vi "NewPower_Current.vi"(7 "testCurrent":dbl, 8 "error in":errorcluster, 9 "Language":T1, 10 "pwrSwitch":refnum<k21>="Power", 11 "power485":refnum<visa-resource-name>="COM3") -> (0 "error out":errorcluster, 1 "switch":bool[](array[boolean]), 2 "Message":string)   [LabVIEW 2015]
doc: "电源地址\n300A大电源，A002\n5A小电源，A001"
uses:
  CustomControl/Lang_Control.ctl
  <vilib>/DAQmx/write.llb/DAQmx Write (Digital 1D Bool NChan 1Samp 1Line).vi
  <vilib>/Instr/_visa.llb/VISA Configure Serial Port (Instr).vi
  <vilib>/DAQmx/miscellaneous.llb/DAQmx Fill In Error Info.vi
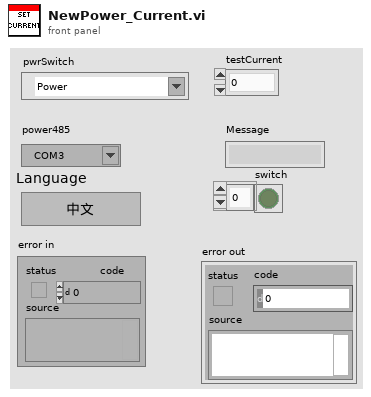
[diagram p1: front panel]
types:
  T1 = typedef "Lang_Control.ctl" = enum16{"中文", "English"}
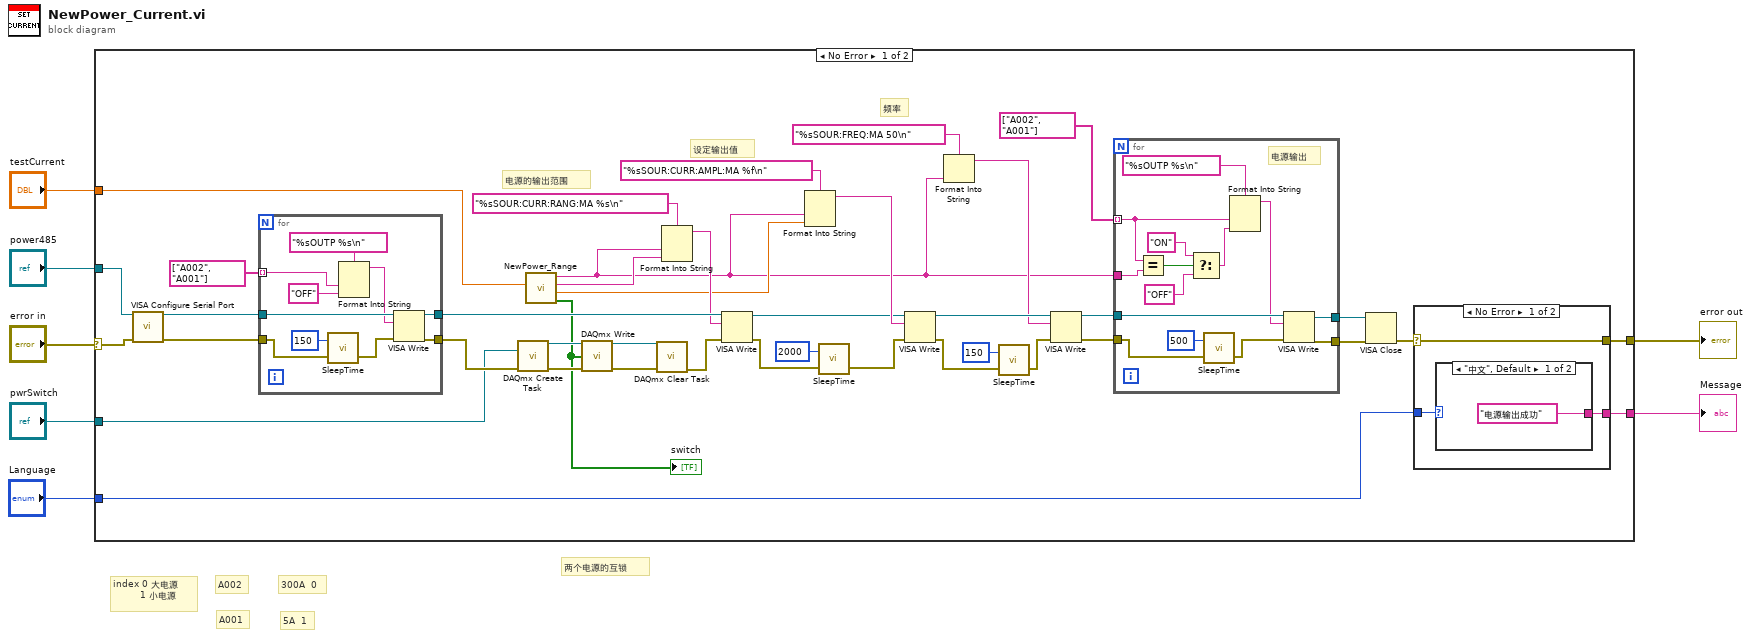
[diagram p0: block diagram]
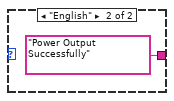
[diagram p2: hidden frame]
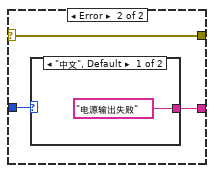
[diagram p3: hidden frame]
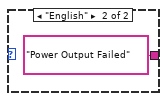
[diagram p4: hidden frame]
diagram:
  # "两个电源的互锁"
  # "index 0 大电源\n         1 小电源"
  # "A001"
  # "A002"
  # "5A  1"
  # "300A  0"
  n1 = case shown="No Error" "error in" {
    selector: "error in" -> [w19 w83]
    tunnel: "power485" -> [w48 _]
    tunnel: "testCurrent" -> [w46 _]
    tunnel: "pwrSwitch" -> [w20 _]
    tunnel: [w17 w83] -> w4
    tunnel: "Language" -> [w16 _]
    tunnel: [w15 _] -> w1
    frame No Error {
      # "频率"
      # "设定输出值"
      # "电源的输出范围"
      n2 = call-poly "VISA Configure Serial Port"("VISA resource name"=w48, "error in (no error)"=w19) -> ("VISA resource name out"=w34:refnum<visa-resource-name>, "error out"=w33:errorcluster)  [unwired: 12 in]
      n3 = for {
        tunnel: w34 -> [w68]
        tunnel: [w67] -> w23
        tunnel: w33 -> [w60]
        tunnel: [w66] -> w32
        tunnel: string[] ["A002", "A001"] -> [w62] mode=indexing
        n4 = call "SleepTime.vi"("error in (no error)"=w60, "Sleep"=u32 150) -> ("error out"=w61:errorcluster)  [unwired: 1 in]
        n5 = Format Into String(format string="%sOUTP %s\n", w62, "OFF" ("format string")) -> (resulting string=w63:string)  [unwired: 2 in, 1 out]
        n6 = VISA Write(VISA resource name=w68, write buffer=w63, error in (no error)=w61) -> (VISA resource name out=w66:refnum<visa-resource-name>, error out=w67:errorcluster)  [unwired: 1 out]
      }
      n7 = call <vilib>:"DAQmx Create Task.vi"("task to copy"=w20, "error in"=w23) -> ("task out"=w38:refnum<k21>, "error out"=w37:errorcluster)  [unwired: 12 in]
      n8 = call "NewPower_Range.vi"("电流值"=w46) -> ("switch"=w21:bool[], "current"=w28:dbl, "region"=w29:string, "adress"=w25:string)  [unwired: 7 in]
      "switch" <- w21
      n9 = call-poly <vilib>:"DAQmx Write.vi"("task/channels in"=w38, "data"=w21, "error in"=w37) -> ("task out"=w35:refnum<k21>, "error out"=w36:errorcluster)  [unwired: 10 in, 1 out]
      n10 = call <vilib>:"DAQmx Clear Task.vi"("task in"=w35, "error in"=w36) -> ("error out"=w22:errorcluster)  [unwired: 13 in]
      n11 = Format Into String(format string="%sSOUR:CURR:RANG:MA %s\n", w25, w29) -> (resulting string=w31:string)  [unwired: 2 in, 1 out]
      n12 = VISA Write(VISA resource name=w32, write buffer=w31, error in (no error)=w22) -> (VISA resource name out=w8:refnum<visa-resource-name>, error out=w14:errorcluster)  [unwired: 1 out]
      n13 = Format Into String(format string="%sSOUR:CURR:AMPL:MA %f\n", w25, w28) -> (resulting string=w30:string)  [unwired: 2 in, 1 out]
      n14 = call "SleepTime.vi"("error in (no error)"=w14, "Sleep"=u32 2000) -> ("error out"=w13:errorcluster)  [unwired: 1 in]
      n15 = VISA Write(VISA resource name=w8, write buffer=w30, error in (no error)=w13) -> (VISA resource name out=w45:refnum<visa-resource-name>, error out=w11:errorcluster)  [unwired: 1 out]
      n16 = Format Into String(format string="%sSOUR:FREQ:MA 50\n", w25) -> (resulting string=w27:string)  [unwired: 2 in, 1 out]
      n17 = call "SleepTime.vi"("error in (no error)"=w11, "Sleep"=u32 150) -> ("error out"=w10:errorcluster)  [unwired: 1 in]
      n18 = VISA Write(VISA resource name=w45, write buffer=w27, error in (no error)=w10) -> (VISA resource name out=w39:refnum<visa-resource-name>, error out=w42:errorcluster)  [unwired: 1 out]
      n19 = for {
        tunnel: w39 -> [w81]
        tunnel: w42 -> [w71]
        tunnel: [w80] -> w41
        tunnel: [w79] -> w40
        tunnel: string[] ["A002", "A001"] -> [w78] mode=indexing
        tunnel: w25 -> [w73]
        # "电源输出"
        n20 = Equal?(x=w78, y=w73) -> (x = y?=w77:bool)
        n21 = Select(t="ON" ("format string"), s=w77, f="OFF" ("format string")) -> (s? t:f=w72:string)
        n22 = call "SleepTime.vi"("error in (no error)"=w71, "Sleep"=u32 500) -> ("error out"=w70:errorcluster)  [unwired: 1 in]
        n23 = Format Into String(format string="%sOUTP %s\n", w78, w72) -> (resulting string=w74:string)  [unwired: 2 in, 1 out]
        n24 = VISA Write(VISA resource name=w81, write buffer=w74, error in (no error)=w70) -> (VISA resource name out=w80:refnum<visa-resource-name>, error out=w79:errorcluster)  [unwired: 1 out]
      }
      n25 = VISA Close(VISA resource name=w41, error in (no error)=w40) -> (error out=w18:errorcluster)
      n26 = case shown="No Error" w18 {
        selector: w18 -> [w51 w56]
        tunnel: [w51 w56] -> w17
        tunnel: w16 -> [w50 w55]
        tunnel: [w49 w54] -> w15
        frame No Error {
          n27 = case shown="\"中文\", Default" w50 {
            tunnel: ["电源输出成功" "Power Output Successfully"] -> w49
            frame "中文", Default {
            }
            frame "English" {
            }
          }
        }
        frame Error {
          n28 = case shown="\"中文\", Default" w55 {
            tunnel: ["电源输出失败" "Power Output Failed"] -> w54
            frame "中文", Default {
            }
            frame "English" {
            }
          }
        }
      }
    }
    frame Error {
    }
  }
  "error out" <- w4
  "Message" <- w1
